vi "DBToString.vi"(1 "Enum":T1) -> (0 "Refname":string)   [LabVIEW 2012]
uses:
  Sally_Dashboard_2013/DBNameEnum.ctl
panel:
  in  "NumCalls":i32[](array[numeric])=[0, 0, 0, 0, 0, 0, 0, 0, 0, 0, 0, 0, 0, 0, 0, 0, 0, 0, 0, 0, 0, 0, 0, 0, 0, 0, 0, 0, 0, 0, 0, 0]
  in  "RefnameArray":string[](array[string])=["AutoInstructions", "DriveLoopTime", "DriveAlignLSLeft", "DriveAlignLSRight", "Use2DriveAlign", "ClimbLS", "LauncherAngleMatches", "FrameworkVision", "sLauncherAngle", "LauncherTargetAngle", "sLauncherRPM", "LauncherTargetRPM", "sDriveDistance", "LauncherMotorValue", "PullbackTol", "FireTol", "LauncherRPMTol", "LauncherAngleTol", "InitialWait", "WaitBetweenLaunch", "AnglePresets", "RPMPresets", "UseAngleEncoder", "UseLauncherEncoder", "UseLauncherPID", "QSWaitBeforeFire", "QSWaitBeforeRetract", "AngleForwardValue", "AngleBackwardValue", "UseClusterArray", "BackupAuto", "ReverseDriveIndicate", "HalfSpeedFactor"]
  # "SET CHANGED VALUES\nAS DEFAULTS!!!"
  # "SET CHANGED VALUES\nAS DEFAULTS!!!"
  # "SET CHANGED VALUES\nAS DEFAULTS!!!"
  # "SET CHANGED VALUES\nAS DEFAULTS!!!"
  # "SET CHANGED VALUES\nAS DEFAULTS!!!"
  # "SET CHANGED VALUES\nAS DEFAULTS!!!"
  # "SET CHANGED VALUES\nAS DEFAULTS!!!"
  # "SET CHANGED VALUES\nAS DEFAULTS!!!"
  # "SET CHANGED VALUES\nAS DEFAULTS!!!"
  # "SET CHANGED VALUES\nAS DEFAULTS!!!"
  # "SET CHANGED VALUES\nAS DEFAULTS!!!"
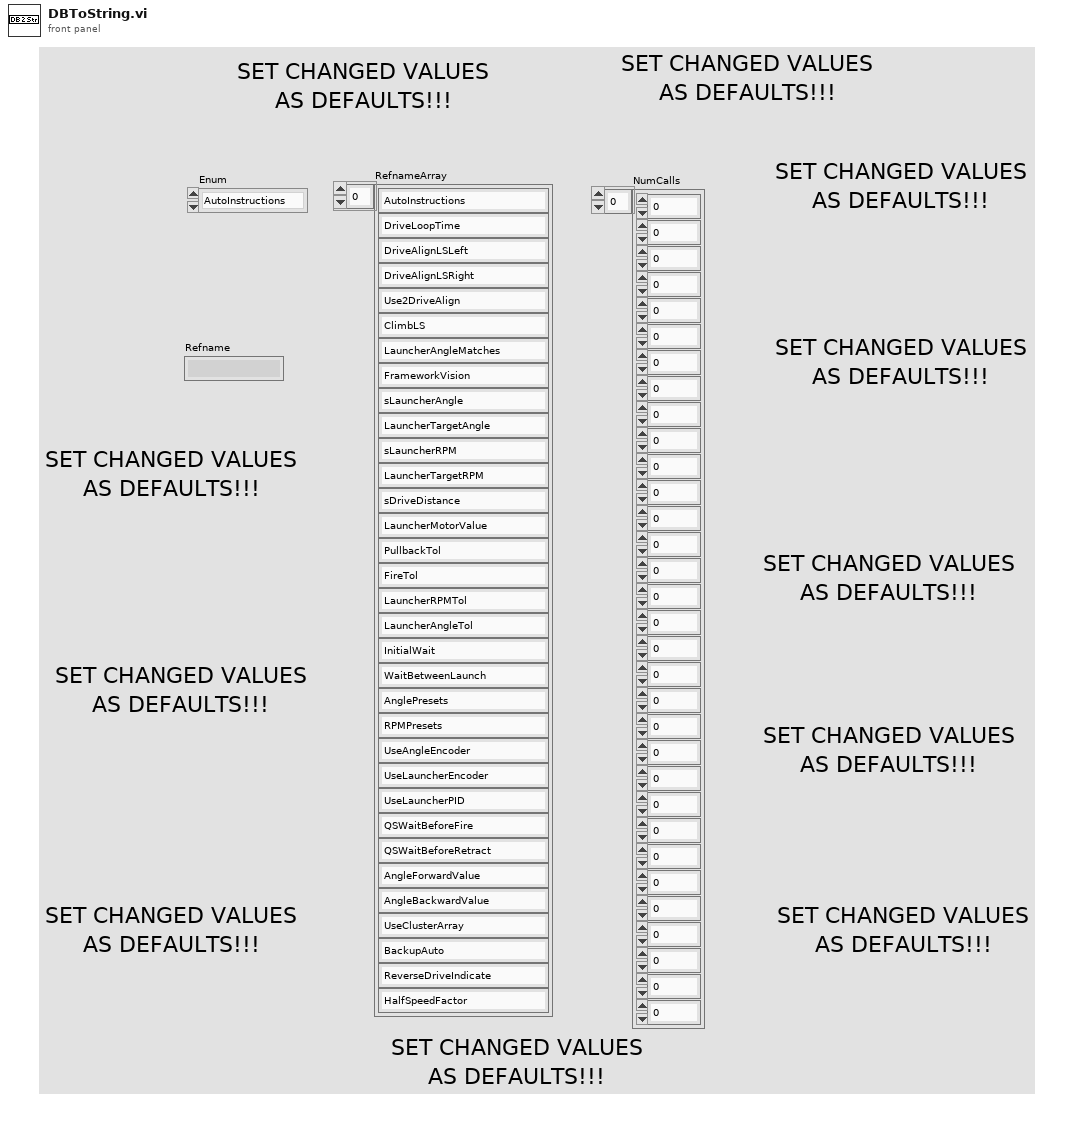
[diagram p1: front panel]
types:
  T1 = typedef "DBNameEnum.ctl" = enum16{"AutoInstructions", "DriveLoopTime", "DriveAlignLSLeft", "DriveAlignLSRight", "Use2DriveAlign", "ClimbLS", "LauncherAngleMatches", "FrameworkVersion", "sLauncherAngle", "LauncherTargetAngle", "sLauncherRPM", "LauncherTargetRPM", "sDriveDistance", "LauncherMotorValue", "PullbackTol", "FireTol", "LauncherRPMTol", "LauncherAngleTol", "InitialWait", "WaitBetweenLaunch", "AnglePresets", "RPMPresets", "UseAngleEncoder", "UseLauncherEncoder", "UseLauncherPID", "QSWaitBeforeFire", "QSWaitBeforeRetract", "AngleForwardValue", "AngleBackwardValue", "UseClusterArray", "BackupAuto", "ReverseDriveIndicate", "HalfSpeedFactor"}
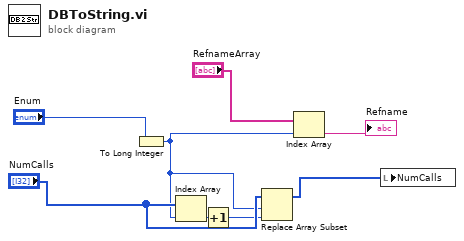
[diagram p0: block diagram]
diagram:
  n1 = To Long Integer(number="Enum") -> (32bit integer=w3:i32)
  n2 = Index Array(array="NumCalls", index=w3) -> (element=w4:i32)
  n3 = Increment(x=w4) -> (x+1=w1:i32)
  n4 = Replace Array Subset(array="NumCalls", new element=w1, index=w3) -> (w2:i32[])
  n5 = Index Array(array="RefnameArray", index=w3) -> (element=→"Refname":string)
  n6 = local write "NumCalls"(w2) -> ()
